vi "FlatToRichsift_proxy_v1_ChannelConfig.vi"(5 "OutputClusterType":T1, 11 "InputCluster":T5) -> (3 "OutputCluster":T1)   [LabVIEW 2024, in "SiftProxy_client.lvlib"]
uses:
  sift_proxy_v1_ChannelConfig_Flat.ctl
  sift_proxy_v1_ChannelDataType.ctl
  sift_proxy_v1_ChannelEnumType_Flat.ctl
  sift_proxy_v1_ChannelBitFieldElement_Flat.ctl
  sift_proxy_v1_ChannelConfig.ctl
  sift_proxy_v1_ChannelEnumType.ctl
  sift_proxy_v1_ChannelBitFieldElement.ctl
  SiftProxy_client.lvlib
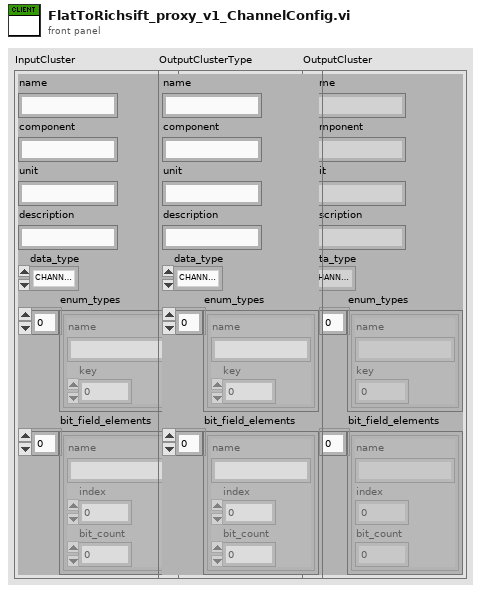
[diagram p1: front panel]
types:
  T1 = typedef "SiftProxy_client.lvlib/sift_proxy_v1_ChannelConfig.ctl" = cluster{"name":string, "component":string, "unit":string, "description":string, "data_type":T2, "enum_types":T3[], "bit_field_elements":T4[]}
  T2 = typedef "SiftProxy_client.lvlib/sift_proxy_v1_ChannelDataType.ctl" = enum32{"CHANNEL_DATA_TYPE_UNSPECIFIED", "CHANNEL_DATA_TYPE_DOUBLE", "CHANNEL_DATA_TYPE_STRING", "CHANNEL_DATA_TYPE_ENUM", "CHANNEL_DATA_TYPE_BIT_FIELD", "CHANNEL_DATA_TYPE_BOOL", "CHANNEL_DATA_TYPE_FLOAT", "CHANNEL_DATA_TYPE_INT_32", "CHANNEL_DATA_TYPE_UINT_32", "CHANNEL_DATA_TYPE_INT_64", "CHANNEL_DATA_TYPE_UINT_64"}
  T3 = typedef "SiftProxy_client.lvlib/sift_proxy_v1_ChannelEnumType.ctl" = cluster{"name":string, "key":u32}
  T4 = typedef "SiftProxy_client.lvlib/sift_proxy_v1_ChannelBitFieldElement.ctl" = cluster{"name":string, "index":i32, "bit_count":u32}
  T5 = typedef "SiftProxy_client.lvlib/sift_proxy_v1_ChannelConfig_Flat.ctl" = cluster{"name":string, "component":string, "unit":string, "description":string, "data_type":T2, "enum_types":T6[], "bit_field_elements":T7[]}
  T6 = typedef "SiftProxy_client.lvlib/sift_proxy_v1_ChannelEnumType_Flat.ctl" = cluster{"name":string, "key":u32}
  T7 = typedef "SiftProxy_client.lvlib/sift_proxy_v1_ChannelBitFieldElement_Flat.ctl" = cluster{"name":string, "index":i32, "bit_count":u32}
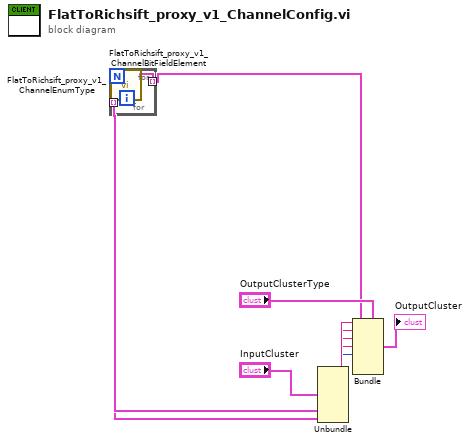
[diagram p0: block diagram]
diagram:
  n1 = Unbundle "Unbundle"("InputCluster") -> ("name"=w9:string, "component"=w8:string, "unit"=w7:string, "description"=w6:string, "data_type"=w5:T2, "enum_types"=w4:T6[], "bit_field_elements"=w2:T7[])
  n2 = for {
    tunnel: w2 -> [w14] mode=indexing
    tunnel: [w13] -> w1 mode=indexing
    n3 = call "FlatToRichsift_proxy_v1_ChannelBitFieldElement.vi"("InputCluster"=w14) -> ("OutputCluster"=w13:T4)  [unwired: 10 in]
  }
  n4 = for {
    tunnel: w4 -> [w16] mode=indexing
    tunnel: [w15] -> w3 mode=indexing
    n5 = call "FlatToRichsift_proxy_v1_ChannelEnumType.vi"("InputCluster"=w16) -> ("OutputCluster"=w15:T3)  [unwired: 10 in]
  }
  n6 = Bundle "Bundle"(cluster="OutputClusterType", "name"=w9, "component"=w8, "unit"=w7, "description"=w6, "data_type"=w5, "enum_types"=w3, "bit_field_elements"=w1) -> (→"OutputCluster":T1)
